vi "Get Temperature Controller Instance ID.vi"(4 "error in (no error)":errorcluster, 6 "Instance Name":T1, 7 "Connection In":refnum<k7>) -> (0 "error out":errorcluster, 2 "tc_id":i32, 3 "Connection Out":refnum<k7>)   [LabVIEW 2020, in "Config Data.lvlib" / "Config Data_DB_ADO.lvclass"]
uses:
  Config Data_DB_ADO.lvclass
  toolbox/ADO Database Drivers/ADO Database Drivers.lvlib
  Startup Processes/_typedefs/Subpanel Names.ctl
  Startup Processes/Startup Processes.lvlib
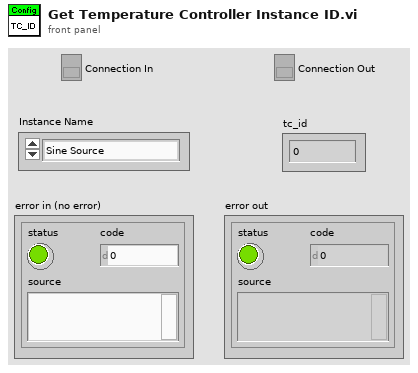
[diagram p1: front panel]
types:
  T1 = typedef "Startup Processes.lvlib/Subpanel Names.ctl" = enum16{"Sine Source", "Ramp Source", "Hen House TC", "Dog House TC", "Out House TC"}
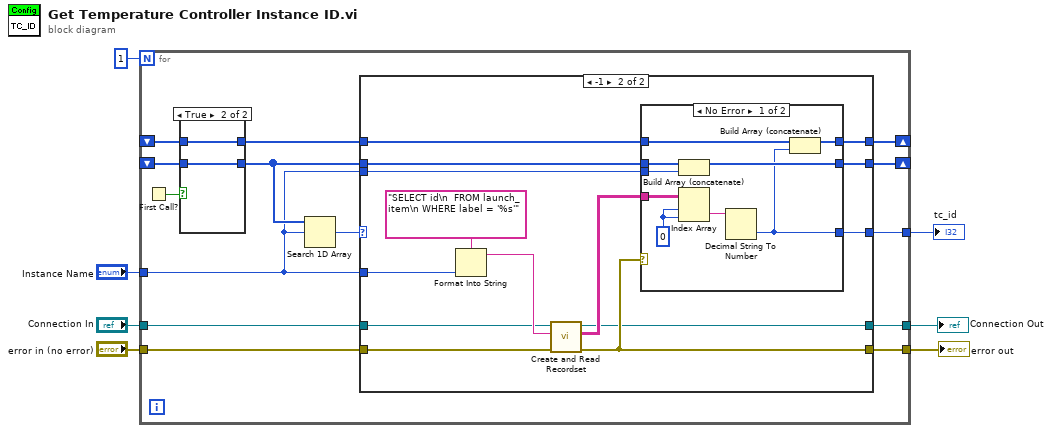
[diagram p0: block diagram]
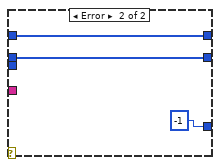
[diagram p3: hidden frame]
diagram:
  n1 = for {
    N: 1 -> [_]
    tunnel: "Instance Name" -> [w10]
    tunnel: [w19] -> w5
    tunnel: "error in (no error)" -> [w21]
    tunnel: [w20] -> w6
    shift-right: [w11] -> _
    shift-left: _ -> [w17]
    shift-right: [w12] -> _
    shift-left: _ -> [w16]
    tunnel: [w9] -> w2
    tunnel: "Connection In" -> [w8]
    n2 = First Call?() -> (First Call?: T/F=w18:bool)
    n3 = case shown="True" w18 {
      tunnel: w17 -> [_ w54]
      tunnel: w16 -> [_ w55]
      tunnel: [_ w55] -> w14
      tunnel: [_ w54] -> w15
      frame False {
      }
      frame True {
      }
    }
    n4 = Search 1D Array(1D array=w15, element=w10) -> (index of element=w13:i32)  [unwired: 1 in]
    n5 = case shown="-1" w13 {
      selector: w13 -> [w25 _]
      tunnel: w21 -> [w26 w31]
      tunnel: [w26 w30] -> w20
      tunnel: [w23 w39] -> w19
      tunnel: w10 -> [_ w37]
      tunnel: w15 -> [w27 w35]
      tunnel: w14 -> [w24 w36]
      tunnel: [w24 w34] -> w12
      tunnel: [w27 w33] -> w11
      tunnel: w10 -> [_ w32]
      tunnel: [w22 w29] -> w9
      tunnel: w8 -> [w22 w28]
      frame Default {
        n6 = Index Array(array=w24, index=w25) -> (element=w23:i32)
      }
      frame -1 {
        n7 = Format Into String(format string="SELECT id\n  FROM launch_item\n WHERE label = '%s'", w37) -> (resulting string=w41:string)  [unwired: 2 in, 1 out]
        n8 = call "Create and Read Recordset.vi"("error in (no error)"=w31, "Source"=w41, "Connection In"=w28) -> ("error out"=w30:errorcluster, "DB Data"=w40:string[][], "Connection Out"=w29:refnum<k7>)  [unwired: 2 in, 2 out]
        n9 = case shown="No Error" w30 {
          tunnel: w40 -> [w50 _]
          tunnel: [w42 -1] -> w39
          tunnel: w36 -> [w44 w53]
          tunnel: w35 -> [w47 w52]
          tunnel: [w43 w53] -> w34
          tunnel: [w46 w52] -> w33
          tunnel: w32 -> [w45 _]
          frame No Error {
            w49 = 0 ("disabled index (col)")
            n10 = Build Array (concatenate)(w47, w45) -> (w46:T1[])
            n11 = Index Array(array=w50, index (row)=w49, index (col)=w49) -> (element=w48:string)
            n12 = Decimal String To Number(string=w48) -> (number=w42:i32)  [unwired: 2 in, 1 out]
            n13 = Build Array (concatenate)(w44, w42) -> (w43:i32[])
          }
          frame Error {
          }
        }
      }
    }
  }
  "tc_id" <- w5
  "error out" <- w6
  "Connection Out" <- w2
